vi "GSI-HVSwitch2.set modified data.vi"(0 "i ref in":refnum<vi>, 2 "i attribute":T1={"SDEX VISA Cluster"={"VISA resource name"="", "HEX address"=0, "VISA Timeout Value (1000 ms)"=1000, "Lock Timeout (1000 ms)"=1000, "semaphore"=refnum, "Baud rate"=0, "revision"=enum."unknown", "deviceInfo"=""}, "SetVoltage SW0"=0.0, "SetVoltage SW1"=0.0, "ActTempAmp"=0.0, "ActTempPS1"=0.0, "ActTempPS2"=0.0, "mode"=enum."unknown", "interfaceInitialized"=FALSE, "serviceIDs"={"nomVoltage0ID"=0, "nomVoltage1ID"=0, "actTempAmpID"=0, "actTempPS1ID"=0, "actTempPS2ID"=0, "modeID"=0}, "usedChannels"=0} {"SDEX VISA Cluster"."HEX address" format="%.0x"}, 5 "error in (no error)":errorcluster) -> (14 "i ref out":refnum<vi>, 19 "error out":errorcluster)   [LabVIEW 2014, in "GSI-HVSwitch2.lvlib"]
doc: "Writes the data into the attribute of an object. Then, the attribute data are unlocked using the \"release\" method. Prior to calling THIS method, the attribute data must have been locked using the methods \"lock\" or \"get data to modify\".\n\n\nLicense Agreement for this software:\n\nCopyright (C)\nGesellschaft für Schwerionenforschung, GSI\nPlanckstr. 1\n64291 Darmstadt\nGermany\n\nContact: D.Beck@gsi.de \n\nThis program is free software; you can redistribute it and/or modify it under the terms of the GNU General Public License as published by the Free Software Foundation; either version 2 of the license, or (at your option) any later version.\n\nThis program is distributed in the hope that it will be useful, but WITHOUT ANY WARRANTY; without even the implied warranty of MERCHANTABILITY or FITNESS FOR A PARTICULAR PURPOSE. See the GNU General License for more details (http://www.gnu.org).\n\nGesellschaft für Schwerionenforschung, GSI\nPlanckstr. 1, 64291 Darmstadt, Germany\nFor all questions and ideas contact: M.Richter@gsi.de, H.Brand@gsi.de or D.Beck@gsi.de.\nLast update: 17-JUN-2004"
uses:
  GSI-HVSwitch2.lvlib
  GSI-HVSwitch2.i attribute.ctl
  CSinstr.lib/SDEX/SDEX.VISA Control.ctl
  CSinstr.lib/SDEX/SDEX.revisionType.ctl
  GSI-HVSwitch2.mode.ctl
  CSCore/CSObj/CSObj.lvlib
  CSinstr.lib/SDEX/SDEXDriver.lvlib
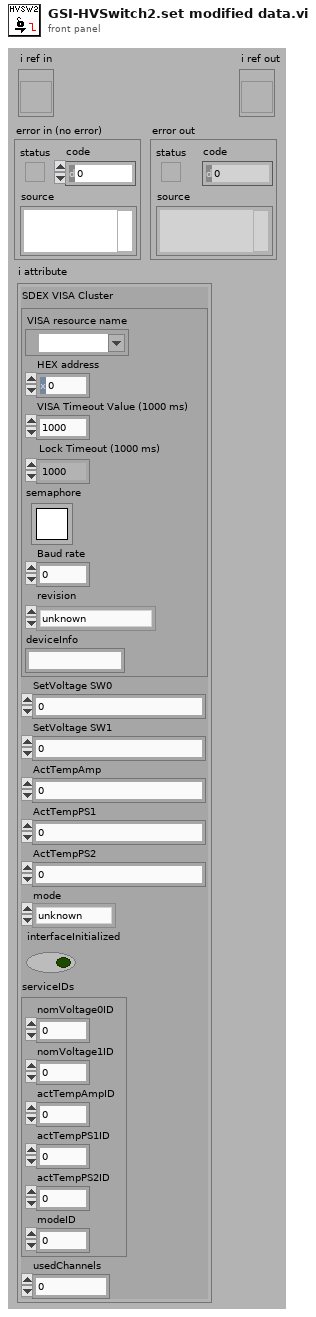
[diagram p1: front panel]
types:
  T1 = typedef "GSI-HVSwitch2.lvlib/GSI-HVSwitch2.i attribute.ctl" = cluster{"SDEX VISA Cluster":T2, "SetVoltage SW0":dbl, "SetVoltage SW1":dbl, "ActTempAmp":dbl, "ActTempPS1":dbl, "ActTempPS2":dbl, "mode":T5, "interfaceInitialized":bool, "serviceIDs":cluster{"nomVoltage0ID":i32, "nomVoltage1ID":i32, "actTempAmpID":i32, "actTempPS1ID":i32, "actTempPS2ID":i32, "modeID":i32}, "usedChannels":i32}
  T2 = typedef "SDEXDriver.lvlib/SDEX.VISA Control.ctl" = cluster{"VISA resource name":refnum<visa-resource-name>, "HEX address":u16, "VISA Timeout Value (1000 ms)":u32, "Lock Timeout (1000 ms)":u32, "semaphore":T3, "Baud rate":u32, "revision":T4, "deviceInfo":string}
  T3 = typedef "Semaphore RefNum" = refnum<k1>
  T4 = typedef "SDEXDriver.lvlib/SDEX.revisionType.ctl" = enum16{"unknown", "hvamp3", "hvswi1", "htrp0", "WDG0"}
  T5 = typedef "GSI-HVSwitch2.lvlib/GSI-HVSwitch2.mode.ctl" = enum16{"unknown", "switch", "stepper"}
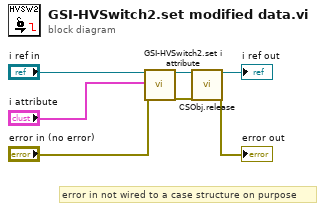
[diagram p0: block diagram]
diagram:
  # "error in not wired to a case structure on purpose"
  n1 = call "GSI-HVSwitch2.set i attribute.vi"("i ref in"="i ref in", "i attribute"="i attribute", "error in (no error)"="error in (no error)") -> ("i ref out"=w4:refnum<vi>, "error out"=w3:errorcluster)  [unwired: 15 in]
  n2 = call "CSObj.release.vi"("i ref in"=w4, "error in (no error)"=w3) -> ("i ref out"=→"i ref out":refnum<vi>, "error out"=→"error out":errorcluster)  [unwired: 16 in]
